vi "Get_Next_Round.vi"(11 "TeamNo":u16) -> (3 "NextRound":u16)   [LabVIEW 2013]
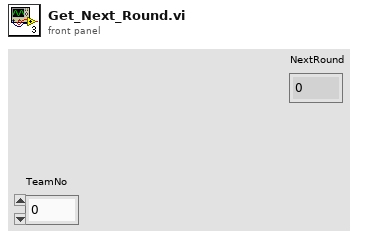
[diagram p1: front panel]
types:
  T1 = typedef "Team Data.ctl" = cluster{"Both":string, "Name":string, "GUID":u16, "Number":u16}
  T2 = typedef "ScoreList.ctl" = cluster{"ValidationCount":u16, "Score":T3}[]
  T3 = typedef "Full Score Entry.ctl" = cluster{"GUID":u16, "Score Mode Selector":u16, "Round Number":u16, "Full Score Entry":T4}
  T4 = typedef "ScoreEntry.ctl" = cluster{"Elements":cluster{"Name":string, "Value":string}[], "Score":dbl}
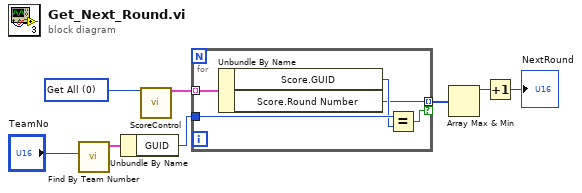
[diagram p0: block diagram]
diagram:
  w7 = u16 0 items=["Get All", "Set", "Reset All", "Force Set", "Force Set All"] ("Get/Set Mode Selector")
  n1 = call "Find By Team Number.vi"("Team Number"="TeamNo") -> ("Team Data"=w5:T1)  [unwired: 9 in, 1 out]
  n2 = Unbundle By Name(w5) -> ("GUID"=w4:u16)
  n3 = call "ScoreControl.vi"("Get/Set Mode Selector"=w7) -> ("Scores"=w6:T2)  [unwired: 13 in, 1 out]
  n4 = for {
    tunnel: w6 -> [w13] mode=indexing
    tunnel: w4 -> [w12]
    tunnel: [w10] -> w3 mode=indexing if=w9
    n5 = Unbundle By Name(w13) -> ("Score.GUID"=w11:u16, "Score.Round Number"=w10:u16)
    n6 = Equal?(x=w12, y=w11) -> (x = y?=w9:bool)
  }
  n7 = Array Max & Min(array=w3) -> (max value=w2:u16)  [unwired: 3 out]
  n8 = Increment(x=w2) -> (x+1=→"NextRound":u16)
